vi "ReadSensor.vi"(1 "World":i8[][](array[numeric])=[[0, 0, 0, 0, 0, 0, 0, 0, 0, 0], [0, 0, 0, 0, 0, 0, 0, 0, 0, 0], [0, 0, 0, 0, 0, 0, 0, 0, 0, 0], [0, 0, 0, 0, 0, 0, 0, 0, 0, 0], [0, 0, 0, 0, 7, 10, 8, 0, 0, 0], [0, 0, 0, 0, 25, 30, 15, 0, 0, 0], [0, 0, 0, 0, 5, 20, 3, 0, 0, 0], [0, 0, 0, 0, 0, 0, 0, 0, 0, 0], [0, 0, 0, 0, 0, 0, 0, 0, 0, 0], [0, 0, 0, 0, 0, 0, 0, 0, 0, 0]], 2 "Y":i8, 3 "X":i8) -> (0 "Sensor Array":i8[][](array[numeric]))   [LabVIEW 2014]
doc: "This VI returns a 3x3 portion of a world array while making sure that it returns correct data when the (X,Y) coordinate asked for is on the edge of the world."
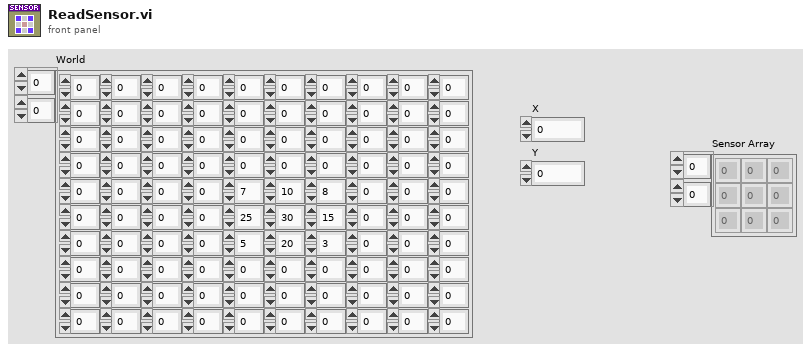
[diagram p1: front panel]
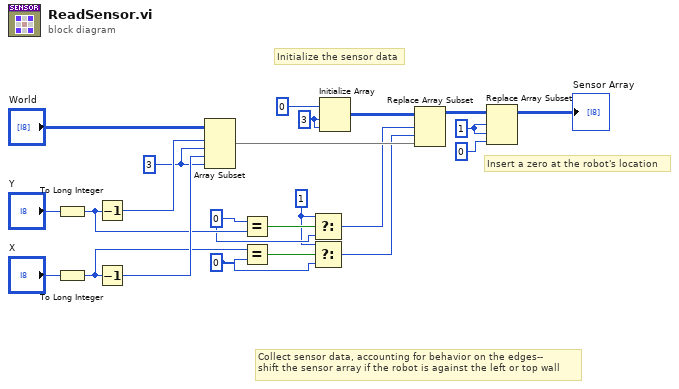
[diagram p0: block diagram]
diagram:
  w1 = 3 ("length")
  w4 = 1 ("index (row)")
  w9 = 3 ("dimension size")
  w11 = 1 ("t")
  w13 = 0 ("y")
  w12 = 0 ("y")
  # "Insert a zero at the robot's location"
  # "Initialize the sensor data"
  # "Collect sensor data, accounting for behavior on the edges--\nshift the sensor array if the robot is against the left or top wall"
  n1 = To Long Integer(number="Y") -> (32bit integer=w16:i32)
  n2 = To Long Integer(number="X") -> (32bit integer=w17:i32)
  n3 = Decrement(x=w16) -> (x-1=w19:i32)
  n4 = Decrement(x=w17) -> (x-1=w18:i32)
  n5 = Array Subset(array="World", index (row)=w19, length (row)=w1, index (col)=w18, length (col)=w1) -> (w23:i8[][])
  n6 = Equal?(x=w13, y=w16) -> (x = y?=w15:bool)
  n7 = Equal?(x=w17, y=w12) -> (x = y?=w14:bool)
  n8 = Select(t=w11, s=w15, f=w13) -> (s? t:f=w10:i32)
  n9 = Select(t=w11, s=w14, f=w12) -> (s? t:f=w6:i32)
  n10 = Initialize Array "Initialize Array"(i8 0 ("element"), w9, w9) -> (w7:i8[][])
  n11 = Replace Array Subset "Replace Array Subset"(array=w7, new element=w23, index (row)=w10, index (col)=w6) -> (w5:i8[][])
  n12 = Replace Array Subset(array=w5, new element=i8 0, index (row)=w4, index (col)=w4) -> (→"Sensor Array":i8[][])
